vi "Agilent34410A Get Errors.vi"(8 "error in (no error)":errorcluster, 11 "VISA Rsrc":refnum<visa-resource-name>="SR530") -> (0 "error out":errorcluster, 3 "VISA Rsrc Out":refnum<visa-resource-name>="GPIB0::12::INSTR", 4 "ChaineRep":string caption="Chaîne de commande")   [LabVIEW 2019]
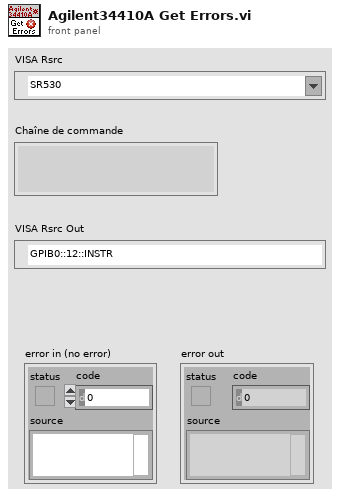
[diagram p1: front panel]
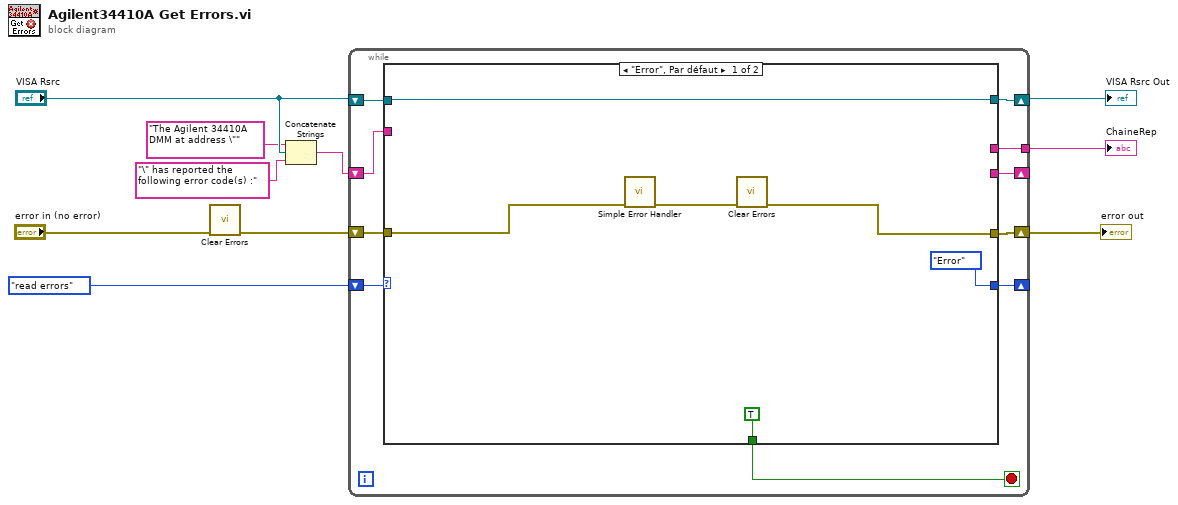
[diagram p0: block diagram]
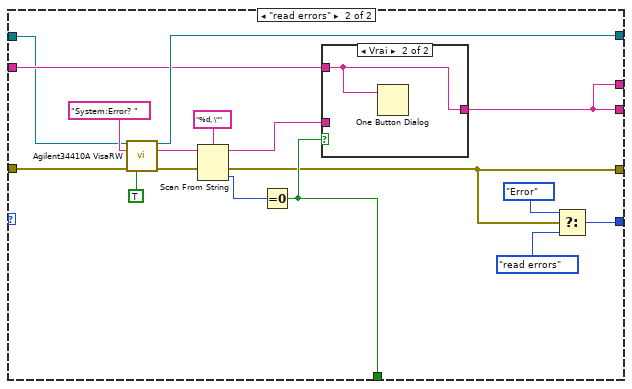
[diagram p2: hidden frame]
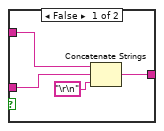
[diagram p3: hidden frame]
diagram:
  n1 = call <vilib>:"Clear Errors.vi"("error in (no error)"="error in (no error)") -> ("error out"=w5:errorcluster)  [unwired: 5 in, 1 out]
  n2 = Concatenate Strings("The Agilent 34410A DMM at address \"" ("string (\"\")"), "VISA Rsrc", "\" has reported the following error code(s) :" ("string (\"\")")) -> (w2:string)
  n3 = while {
    tunnel: [w18] -> w7
    shift-right: [w16] -> w9
    shift-left: w5 -> [w19]
    shift-right: [w20] -> w8
    shift-left: "VISA Rsrc" -> [w11]
    shift-right: [w15] -> _
    shift-left: enum16{"Error", "read errors"}."read errors" -> [w14]
    shift-right: [w13] -> _
    shift-left: w2 -> [w12]
    stop <- w17 stop-if-true
    n4 = case shown="\"Error\", Par défaut" w14 {
      tunnel: [w21 w43] -> w20
      tunnel: w19 -> [w25 w40]
      tunnel: [_ w27] -> w18
      tunnel: [TRUE w31] -> w17
      tunnel: [w22 w28] -> w16
      tunnel: [enum16{"Error", "read errors"}."Error" w34] -> w15
      tunnel: [_ w27] -> w13
      tunnel: w12 -> [_ w33]
      tunnel: w11 -> [w21 w30]
      frame "Error", Default {
        n5 = call <vilib>:"Simple Error Handler.vi"("error in (no error)"=w25) -> ("error out"=w23:errorcluster)  [unwired: 4 in, 4 out]
        n6 = call <vilib>:"Clear Errors.vi"("error in (no error)"=w23) -> ("error out"=w22:errorcluster)  [unwired: 5 in, 1 out]
      }
      frame "read errors" {
        n7 = call <userlib>:"Agilent34410A VisaRW.vi"("VISA Rsrc"=w30, "ChaineCom"="System:Error? " ("string (\"\")"), "error in (no error)"=w40, "Lecture?(T)"=TRUE) -> ("VISA Rsrc Out"=w43:refnum<visa-resource-name>, "ChaineRep"=w29:string, "error out"=w39:errorcluster)  [unwired: 7 in, 2 out]
        n8 = Scan From String(format string="%d, \"" ("chaîne de format"), input string=w29, error in=w39) -> (remaining string=w32:string, error out=w28:errorcluster, output 1=w37:i32)  [unwired: 2 in, 1 out]
        n9 = Equal To 0?(x=w37) -> (x = 0?=w31:bool)
        n10 = case shown="Vrai" w31 {
          tunnel: [w47 w48] -> w27
          tunnel: w33 -> [w46 w48]
          tunnel: w32 -> [w44 _]
          frame False {
            n11 = Concatenate Strings(w46, w44, "\r\n") -> (w47:string)
          }
          frame True {
            n12 = One Button Dialog(message=w48) -> ()  [unwired: 1 in, 1 out]
          }
        }
        n13 = Select(t=enum16{"Error", "read errors"}."Error", s=w28, f=enum16{"Error", "read errors"}."read errors") -> (s? t:f=w34:enum16{"Error", "read errors"})
      }
    }
  }
  "error out" <- w9
  "VISA Rsrc Out" <- w8
  "ChaineRep" <- w7
